vi "CAENHV Set Ch Name.vi"(6 "ChName":string, 7 "ChNum":u16, 8 "error in (no error)":errorcluster, 9 "ChList":u16[](array[numeric]), 10 "slot":u16, 11 "handle":i32) -> (0 "error out":errorcluster)   [LabVIEW 2018, in "CAENHVWrapper.lvlib"]
doc: "CAENHVLIB_API CAENHVRESULT CAENHV_SetChName(int handle, ushort slot, \n ushort ChNum, const ushort *ChList, const char *ChName);"
uses:
  <instrlib>/CAENHVWrapper/CAENHVWrapper.lvlib
  <instrlib>/CAENHVWrapper/VIs/CAENHVWrapper.dll
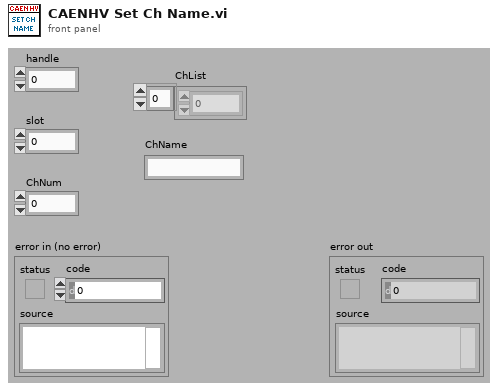
[diagram p1: front panel]
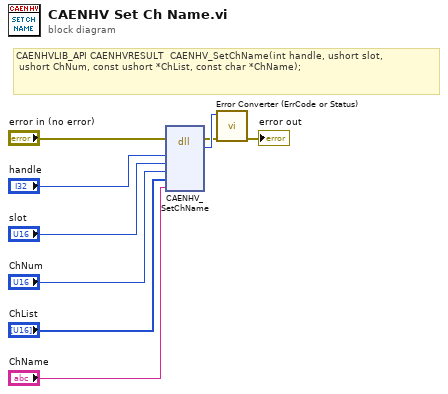
[diagram p0: block diagram]
diagram:
  # "CAENHVLIB_API CAENHVRESULT  CAENHV_SetChName(int handle, ushort slot, \n ushort ChNum, const ushort *ChList, const char *ChName);"
  n1 = dll-call lib="C:/Program Files (x86)/National Instruments/LabVIEW 2018/instr.lib/CAENHVWrapper/VIs/CAENHVWrapper.*" fn="CAENHV_SetChName"(error in="error in (no error)", "handle"="handle", "slot"="slot", "ChNum"="ChNum", "ChList"="ChList", "ChName"="ChName") -> (error out=w4:errorcluster, "return type"=w5:i32)  [unwired: 7 in, 1 out]
  n2 = call <instrlib>:"Error Converter (ErrCode or Status).vi"("error in (no error)"=w4, "error code"=w5) -> ("error out"=→"error out":errorcluster)  [unwired: 9 in]
